vi "Autonomous Independent.vi"() -> ()   [LabVIEW 2016]
doc: "This VI is called when autonomous begins, and will automatically be terminated when autonomous ends. You can carry out timed or sensor driven robot movement independently without needing to return to the caller."
panel:
  in  "Test":T1(ring)=enum."PurePursuit"
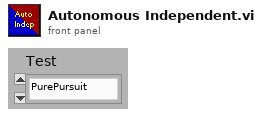
[diagram p1: front panel]
types:
  T1 = enum16{"Straight", "Point", "Swing", "PurePursuit"}
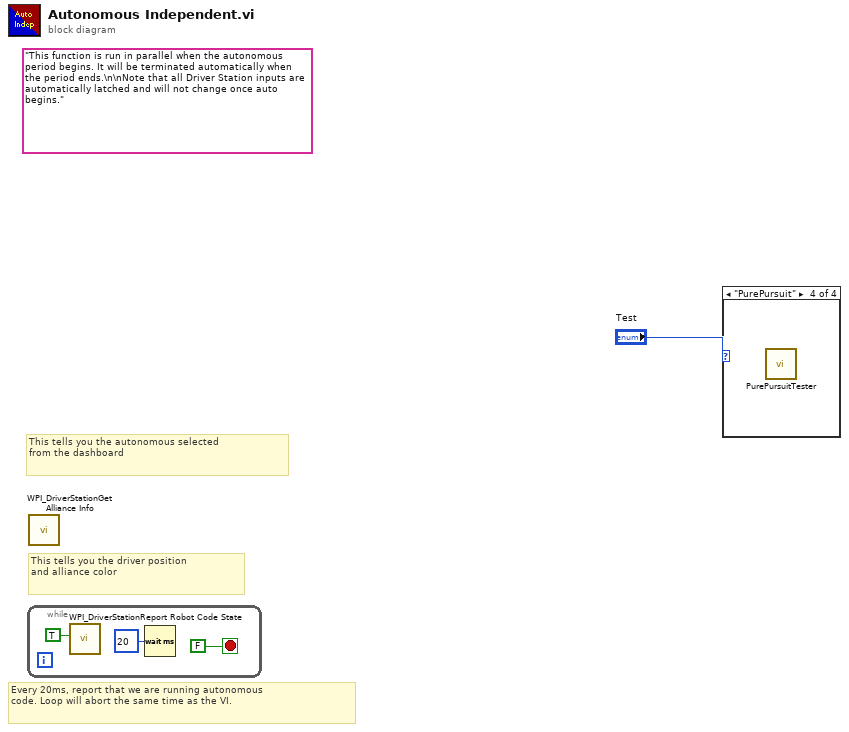
[diagram p0: block diagram]
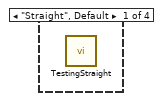
[diagram p2: hidden frame]
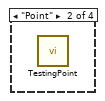
[diagram p3: hidden frame]
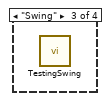
[diagram p4: hidden frame]
diagram:
  (unwired) "This function is run in parallel when the autonomous period begins. It will be terminated automatically when the period ends.\n\nNote that all Driver Station inputs are automatically latched and will not change once auto begins."
  # "This tells you the autonomous selected\nfrom the dashboard"
  # "Every 20ms, report that we are running autonomous\ncode. Loop will abort the same time as the VI."
  # "This tells you the driver position\nand alliance color"
  n1 = while {
    stop <- FALSE stop-if-true
    n2 = call <vilib>:"WPI_DriverStationReport Robot Code State.vi"("Autonomous"=TRUE) -> ()  [unwired: 10 in, 1 out]
    n3 = Wait (ms)(milliseconds to wait=u32 20) -> ()  [unwired: 1 out]
  }
  n4 = call <vilib>:"WPI_DriverStationGet Alliance Info.vi"() -> ()  [unwired: 12 out]
  n5 = case shown="\"PurePursuit\"" "Test" {
    frame "Straight", Default {
      n6 = call "TestingStraight.vi"() -> ()  [unwired: 12 in]
    }
    frame "Point" {
      n7 = call "TestingPoint.vi"() -> ()  [unwired: 12 in]
    }
    frame "Swing" {
      n8 = call "TestingSwing.vi"() -> ()  [unwired: 12 in]
    }
    frame "PurePursuit" {
      n9 = call "PurePursuitTester.vi"() -> ()  [unwired: 12 in]
    }
  }
